vi "Conv_Pounds_Killograms.vi"(10 "Pounds":dbl) -> (2 "Killograms":dbl)   [LabVIEW 2019, in "Trajectory_Library.lvlib"]
doc: "Convert mass in pounds to kilograms\n\nInput:\n - pounds -- mass in pounds\n\nOutput:\n - kilograms -- mass in kilograms"
uses:
  Trajectory_Library.lvlib
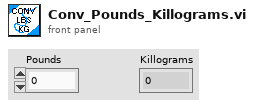
[diagram p1: front panel]
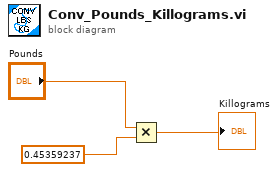
[diagram p0: block diagram]
diagram:
  n1 = Multiply(x="Pounds", y=0.45359237) -> (x*y=→"Killograms":dbl)
